vi "gfitsio-get-variant-info.vi"(8 "error in (no error)":errorcluster, 11 "variant":variant) -> (0 "error out":errorcluster, 1 "data out":u8[](array[numeric]), 2 "cfitsio datatype":T1=1 items=["TBIT"=1, "TBYTE  (U8)"=11, "TSBYTE  (I8)"=12, "TLOGICAL"=14, "TSTRING"=16, "TUSHORT  (U16)"=20, "TSHORT  (I16)"=21, "TUINT"=31, "TULONG  (U32)"=40, "TLONG  (I32)"=41, "TFLOAT  (SGL)"=42, "TLONGLONG  (I64)"=81, "TDOUBLE  (DBL)"=82, "TCOMPLEX  (CSG)"=83, "TDOUBLECOMPLEX  (CDB)"=163], 3 "sizes":i32[](array[numeric]))   [LabVIEW 2013, in "gfitsio.lvlib"]
doc: "Extract the data of a variant as a flattened string (in the form of a U8 1D array because this is easier to pass back and forth with a DLL). Also get the diminsionality of the data in the variant if it is an array or string as well as the base datatype. Report errors if something is passed in the variant incompatible with FITS."
uses:
  gfitsio.lvlib
  cfitsio-datatypes.ctl
  <vilib>/Utility/VariantDataType/VariantType.lvlib
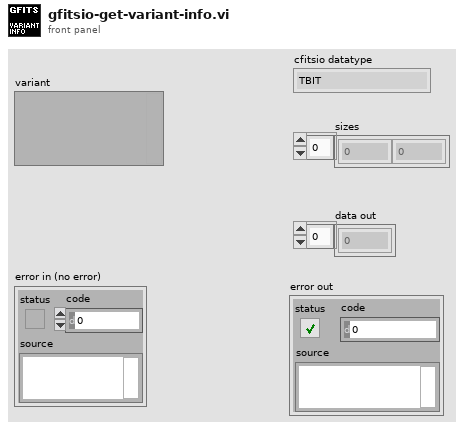
[diagram p1: front panel]
types:
  T1 = typedef "gfitsio.lvlib/cfitsio-datatypes.ctl" = i32
  T2 = enum16{"big-endian, network order", "native, host order", "little-endian"}
  T3 = typedef "VariantType.lvlib/Type.ctl" = enum8{"Invalid Type", "Void", "I8", "I16", "I32", "I64", "U8", "U16", "U32", "U64", "Single Float", "Double Float", "Extended Float", "Single Complex", "Double Complex", "Extended Complex", "Enum U8", "Enum U16", "Enum U32", "Enum U64", "Single Float With Unit", "Double Float With Unit", "Extended Float With Unit", "Single Complex with Unit", "Double Complex with Unit", "Extended Complex with Unit", "Boolean", "String", "Path", "Picture", "Tag", "Array", "Cluster", "Variant", "LV Variant", "Waveform", "Timestamp", "Digital Waveform", "Digital Data", "ExpressData", "Refnum", "External Data", "VI", "Poly VI", "LabVIEW Class Instance", "Fixed Point"}
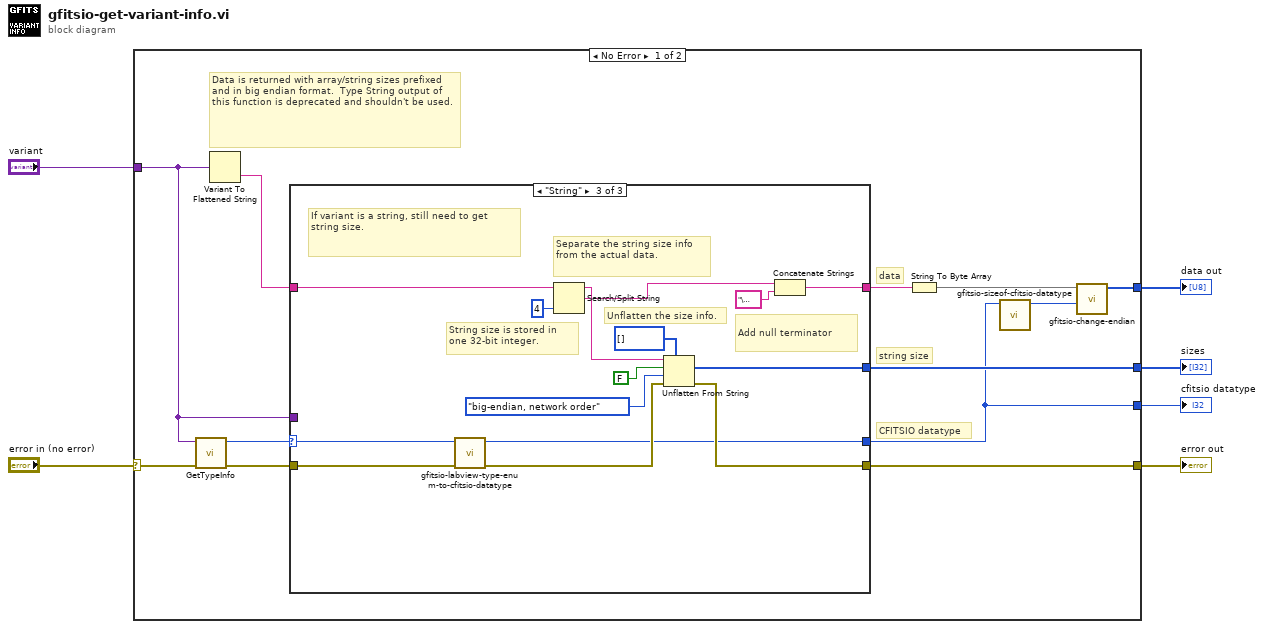
[diagram p0: block diagram]
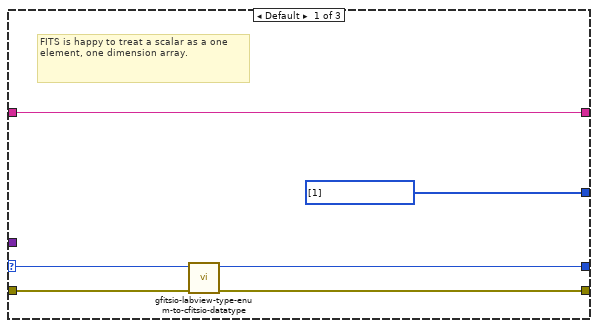
[diagram p2: hidden frame]
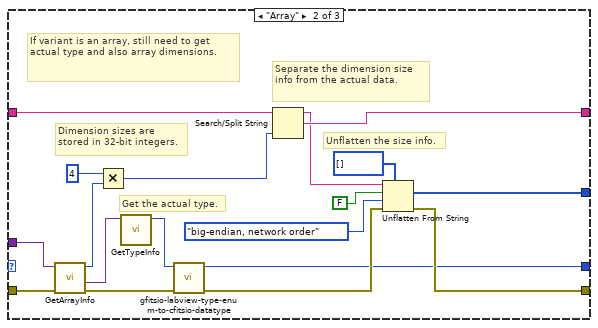
[diagram p3: hidden frame]
diagram:
  n1 = case shown="No Error" "error in (no error)" {
    selector: "error in (no error)" -> [w7 w58]
    tunnel: [w12 _] -> w6
    tunnel: [w11 _] -> w5
    tunnel: "variant" -> [w10 _]
    tunnel: [w9 _] -> w3
    tunnel: [w8 w58] -> w2
    frame No Error {
      # "CFITSIO datatype"
      # "string size"
      # "data"
      # "Data is returned with array/string sizes prefixed and in big endian format.  Type String output of this function is deprecated and shouldn't be used."
      n2 = call <vilib>:"GetTypeInfo.vi"("error in (no error)"=w7, "Variant"=w10) -> ("error out"=w17:errorcluster, "Type Enum"=w18:T3)  [unwired: 5 in, 3 out]
      n3 = Variant To Flattened String(Variant=w10) -> (data string=w16:string)  [unwired: 1 out]
      n4 = case shown="\"String\"" w18 {
        selector: w18 -> [w22 _ w50]
        tunnel: [w21 w25 w51] -> w9
        tunnel: w10 -> [_ w42 _]
        tunnel: w17 -> [w20 w40 w49]
        tunnel: [w19 w30 w53] -> w8
        tunnel: w16 -> [w24 w39 w45]
        tunnel: [w24 w38 w44] -> w15
        tunnel: [i32[] [1] w29 w43] -> w12
        frame Default {
          # "FITS is happy to treat a scalar as a one element, one dimension array."
          n5 = call "gfitsio-labview-type-enum-to-cfitsio-datatype.vi"("error in (no error)"=w20, "LabVIEW Type Enum"=w22) -> ("error out"=w19:errorcluster, "cfitsio datatype"=w21:T1)  [unwired: 8 in]
        }
        frame "Array" {
          # "Get the actual type."
          # "Unflatten the size info."
          # "Separate the dimension size info from the actual data."
          # "Dimension sizes are stored in 32-bit integers."
          # "If variant is an array, still need to get actual type and also array dimensions."
          n6 = call <vilib>:"GetArrayInfo.vi"("error in (no error)"=w40, "Variant"=w42) -> ("error out"=w28:errorcluster, "ArrayElement"=w41:variant, "NDims"=w37:i32)  [unwired: 6 in, 1 out]
          n7 = Multiply(x=4, y=w37) -> (x*y=w35:i32)
          n8 = call <vilib>:"GetTypeInfo.vi"("Variant"=w41) -> ("Type Enum"=w26:T3)  [unwired: 6 in, 4 out]
          n9 = call "gfitsio-labview-type-enum-to-cfitsio-datatype.vi"("error in (no error)"=w28, "LabVIEW Type Enum"=w26) -> ("error out"=w27:errorcluster, "cfitsio datatype"=w25:T1)  [unwired: 8 in]
          n10 = Search/Split String(string=w39, offset (0)=w35) -> (substring before match=w34:string, match + rest of string=w38:string)  [unwired: 1 in, 1 out]
          n11 = Unflatten From String(type=i32[] [], binary string=w34, data includes array or string size? (T)=FALSE, byte order (0:big-endian, network order)=T2."big-endian, network order", error in (no error)=w27) -> (value=w29:i32[], error out=w30:errorcluster)  [unwired: 1 out]
        }
        frame "String" {
          # "Add null terminator"
          # "Unflatten the size info."
          # "Separate the string size info from the actual data."
          # "String size is stored in one 32-bit integer."
          # "If variant is a string, still need to get string size."
          n12 = call "gfitsio-labview-type-enum-to-cfitsio-datatype.vi"("error in (no error)"=w49, "LabVIEW Type Enum"=w50) -> ("error out"=w52:errorcluster, "cfitsio datatype"=w51:T1)  [unwired: 8 in]
          n13 = Search/Split String(string=w45, offset (0)=4 ("x")) -> (substring before match=w57:string, match + rest of string=w47:string)  [unwired: 1 in, 1 out]
          n14 = Unflatten From String(type=i32[] [], binary string=w57, data includes array or string size? (T)=FALSE, byte order (0:big-endian, network order)=T2."big-endian, network order", error in (no error)=w52) -> (value=w43:i32[], error out=w53:errorcluster)  [unwired: 1 out]
          n15 = Concatenate Strings(w47, "\u0000" ("string")) -> (w44:string)
        }
      }
      n16 = String To Byte Array(string=w15) -> (unsigned byte array=w13:u8[])
      n17 = call "gfitsio-sizeof-cfitsio-datatype.vi"("cfitsio datatype"=w9) -> ("size (bytes)"=w14:i32)  [unwired: 8 in, 2 out]
      n18 = call "gfitsio-change-endian.vi"("word size (bytes)"=w14, "data in"=w13) -> ("data out"=w11:u8[])  [unwired: 9 in]
    }
    frame Error {
    }
  }
  "error out" <- w2
  "sizes" <- w6
  "data out" <- w5
  "cfitsio datatype" <- w3
